vi "createXLSX.vi"(8 "error in (no error)":errorcluster, 11 "MS-Excel in":refnum<class "MS-Excel.lvclass">) -> (0 "error out":errorcluster, 3 "MS-Excel out":refnum<class "MS-Excel.lvclass">)   [LabVIEW 2017, in "LabVIEW NPOI.lvlib" / "MS-Excel.lvclass"]
uses:
  MS-Excel.lvclass
  C:/Users/Neo/Desktop/Dev_Tools_BR/LabVIEW_NPOI/src/LabVIEW NPOI/Document/Document.lvclass
  Document/Document.lvclass/Document.ctl
  C:/Program Files (x86)/National Instruments/LabVIEW 2017/vi.lib/BenjaminR/LabVIEW NPOI/lib/NPOI 2.1.1/NPOI.OOXML.dll
  Program Files (x86)/National Instruments/LabVIEW 2017/vi.lib/BenjaminR/LabVIEW NPOI/lib/NPOI 2.1.1/NPOI.OOXML.dll
  Document/Get FilePath.vi
  Support/File Stream/File Stream.lvlib
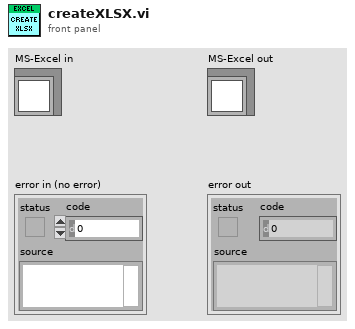
[diagram p1: front panel]
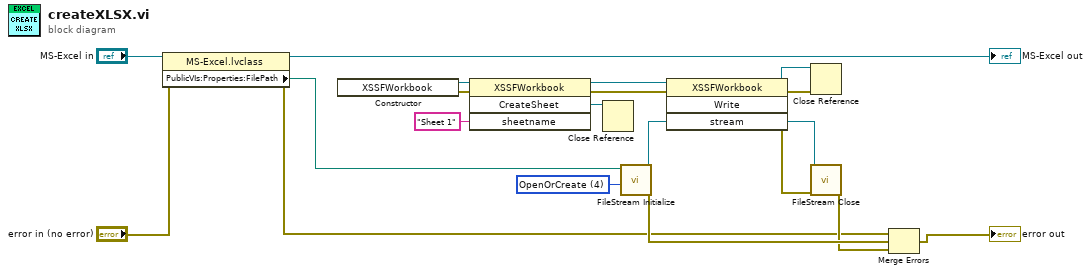
[diagram p0: block diagram]
diagram:
  w8 = 4 items=["CreateNew"=1, "Create"=2, "Open"=3, "OpenOrCreate"=4, "Truncate"=5, "Append"=6] ("mode")
  n1 = property class="MS-Excel.lvclass"(reference="MS-Excel in", error in="error in (no error)") -> (reference out=→"MS-Excel out":refnum<class "MS-Excel.lvclass">, error out=w15:errorcluster, "PublicVIs:Properties:FilePath"=w7:path)
  n2 = constructor class="XSSFWorkbook"() -> (reference out=w6:refnum<k24>, error out=w4:errorcluster)  [unwired: 3 in, 1 out]
  n3 = invoke class="XSSFWorkbook" method="CreateSheet"(reference=w6, error in=w4, "sheetname"="Sheet 1") -> (reference out=w5:refnum<k24>, error out=w3:errorcluster, "CreateSheet"=w2:refnum<k24>)  [unwired: 1 in, 1 out]
  n4 = Close Reference(reference=w2) -> ()  [unwired: 1 in, 1 out]
  n5 = call "FileStream Initialize.vi"("mode"=w8, "path"=w7) -> ("error out"=w17:errorcluster, "new reference"=w18:refnum<k24>)  [unwired: 8 in]
  n6 = invoke class="XSSFWorkbook" method="Write"(reference=w5, error in=w3, "stream"=w18) -> (reference out=w9:refnum<k24>, error out=w10:errorcluster)  [unwired: 1 in, 2 out]
  n7 = Close Reference(reference=w9, error in (no error)=w10) -> ()  [unwired: 1 out]
  n8 = call "FileStream Close.vi"("error in (no error)"=w10, "reference"=w18) -> ("error out"=w16:errorcluster)  [unwired: 9 in]
  n9 = Merge Errors(w15, w17, w16) -> (→"error out":errorcluster)
